vi "Log Header Data.vi"(8 "error in (no error)":errorcluster, 10 "Header Data":string, 11 "Logging Configuration in":T1) -> (0 "error out":errorcluster, 3 "Logging Configuration out":T1)   [LabVIEW 2018, in "Logging.lvlib"]
doc: "This VI uses the TDMS Write function to write data to a TDMS file."
uses:
  Logging.lvlib
  Logging Configuration.ctl
  <vilib>/addons/database/Connection.llb/Conn ObjectReference.ctl
  <vilib>/addons/database/NI_Database_API.lvlib
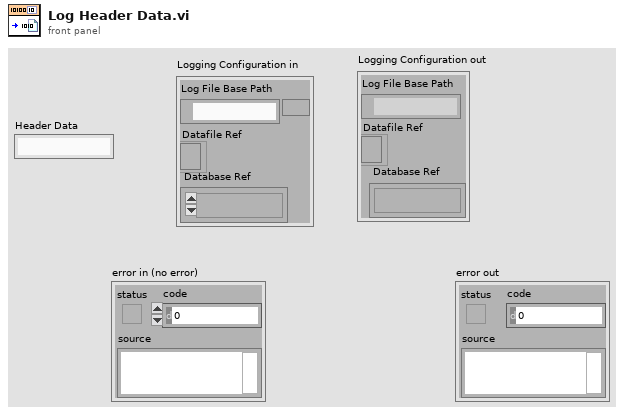
[diagram p1: front panel]
types:
  T1 = typedef "Logging.lvlib/Logging Configuration.ctl" = cluster{"Log File Base Path":path, "Datafile Ref":refnum<file>, "Database Ref":T2}
  T2 = typedef "NI_Database_API.lvlib/Conn ObjectReference.ctl" = refnum<k1>
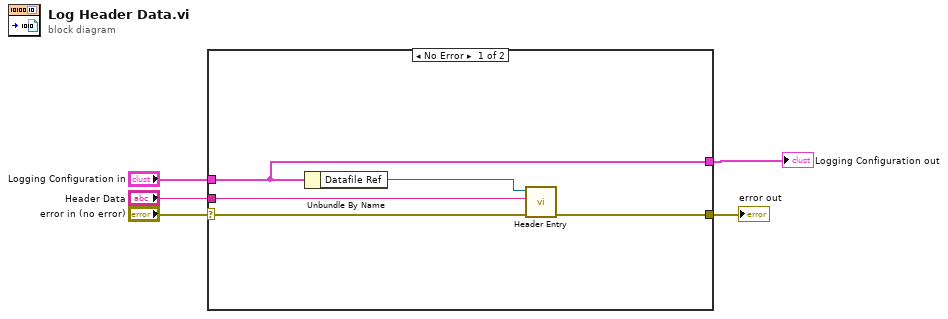
[diagram p0: block diagram]
diagram:
  n1 = case shown="No Error" "error in (no error)" {
    selector: "error in (no error)" -> [w10 w12]
    tunnel: "Logging Configuration in" -> [w6 w11]
    tunnel: [w8 w12] -> w4
    tunnel: "Header Data" -> [w7 _]
    tunnel: [w6 w11] -> w1
    frame No Error {
      n2 = Unbundle By Name(w6) -> ("Datafile Ref"=w9:refnum<file>)
      n3 = call "Header Entry.vi"("error in (no error)"=w10, "Header Data"=w7, "Byte Stream File in"=w9) -> ("error out"=w8:errorcluster)  [unwired: 7 in, 1 out]
    }
    frame Error {
    }
  }
  "error out" <- w4
  "Logging Configuration out" <- w1
